vi "Write Name.vi"(8 "error in":errorcluster, 10 "Name":string, 11 "Property in":refnum<class "Property.lvclass">) -> (0 "error out":errorcluster, 3 "Property out":refnum<class "Property.lvclass">)   [LabVIEW 2024, in "Parser.lvlib" / "Property.lvclass"]
uses:
  Property.lvclass
  Property.lvclass/Property.ctl
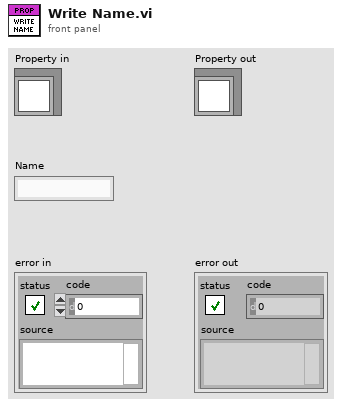
[diagram p1: front panel]
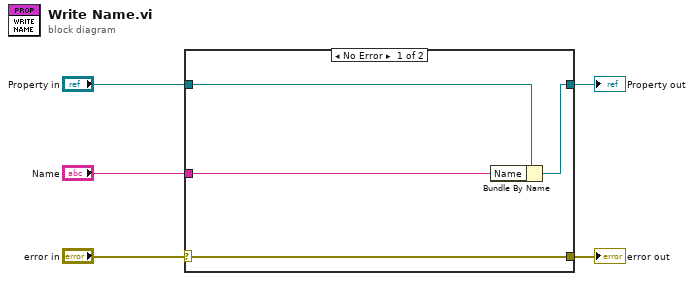
[diagram p0: block diagram]
diagram:
  n1 = case shown="No Error" "error in" {
    selector: "error in" -> [w9 w11]
    tunnel: [w9 w11] -> w4
    tunnel: [w7 w10] -> w2
    tunnel: "Property in" -> [w8 w10]
    tunnel: "Name" -> [w6 _]
    frame No Error {
      n2 = Bundle By Name(cluster=w8, "Name"=w6) -> (w7:refnum<class "Property.lvclass">)
    }
    frame Error {
    }
  }
  "error out" <- w4
  "Property out" <- w2
